vi "Inst.KH7008.setChannel.vi"(8 "error in (no error)":errorcluster, 10 "channelProperties":T1={"channel"=1, "gain"=enum."10", "input"=enum."SE+", "shunt"=enum."50", "couple"=enum."DC", "filter"=enum."ON"} {"channel" min=1 max=8 step=1}, 11 "Inst.Krohn-Hite-7008 in":refnum<class "Inst.Krohn-Hite-7008.lvclass">) -> (0 "error out":errorcluster, 3 "Inst.Krohn-Hite-7008 out":refnum<class "Inst.Krohn-Hite-7008.lvclass">)   [LabVIEW 2019, in "Inst.KH7008.lvlib" / "Inst.Krohn-Hite-7008.lvclass"]
uses:
  Inst.Krohn-Hite-7008.lvclass
  KH7008/typedefs/channelProperties--Cluster.ctl
  KH7008/typedefs/channel--numeric.ctl
  KH7008/typedefs/gain--enum.ctl
  KH7008/typedefs/Input--Enum.ctl
  KH7008/typedefs/shunt--enum.ctl
  KH7008/typedefs/couple--Enum.ctl
  KH7008/typedefs/Filter--Enum.ctl
  Typedefs/setChannelRequest--Cluster.ctl
  KH7008/KH7008.lvlib
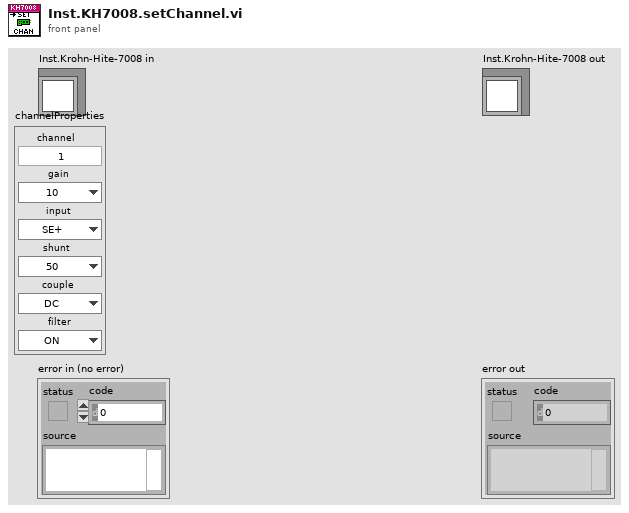
[diagram p1: front panel]
types:
  T1 = typedef "KH7008.lvlib/channelProperties--Cluster.ctl" = cluster{"channel":T2, "gain":T3, "input":T4, "shunt":T5, "couple":T6, "filter":T7}
  T2 = typedef "KH7008.lvlib/channel--numeric.ctl" = u16
  T3 = typedef "KH7008.lvlib/gain--enum.ctl" = enum16{"1", "10", "100", "1000"}
  T4 = typedef "KH7008.lvlib/input--enum.ctl" = enum16{"OFF", "SE+", "SE-", "DIFF"}
  T5 = typedef "KH7008.lvlib/shunt--enum.ctl" = enum16{"Open", "50", "500", "5k", "50k", "10M"}
  T6 = typedef "KH7008.lvlib/couple--enum.ctl" = enum16{"AC", "DC"}
  T7 = typedef "KH7008.lvlib/filter--enum.ctl" = enum16{"OFF", "ON"}
  T8 = typedef "Inst.KH7008.lvlib/Inst.Krohn-Hite-7008.lvclass/setChannelRequest--Cluster.ctl" = cluster{"channelProperties":T1}
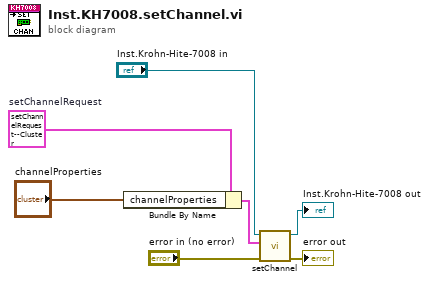
[diagram p0: block diagram]
diagram:
  w7 = T8 {"channelProperties"={"channel"=1, "gain"=enum."10", "input"=enum."OFF", "shunt"=enum."10M", "couple"=enum."AC", "filter"=enum."OFF"}}  # setChannelRequest
  n1 = Bundle By Name(cluster=w7, "channelProperties"="channelProperties") -> (w1:T8)
  n2 = call-dynamic "setChannel.vi"("error in (no error)"="error in (no error)", "channelProperties"=w1, "Inst.Krohn-Hite-7008 in"="Inst.Krohn-Hite-7008 in") -> ("error out"=→"error out":errorcluster, "Inst.Krohn-Hite-7008 out"=→"Inst.Krohn-Hite-7008 out":refnum<class "Inst.Krohn-Hite-7008.lvclass">)  [unwired: 7 in]
